vi "Write resource name.vi"(8 "error in (no error)":errorcluster, 10 "RIO Device":T1, 11 "FPGATarget in":refnum<class "FPGATarget.lvclass">) -> (0 "error out":errorcluster, 3 "FPGATarget out":refnum<class "FPGATarget.lvclass">)   [LabVIEW 2013, in "FPGATarget.lvclass"]
uses:
  FPGATarget.lvclass
  <vilib>/userdefined/High Color/nirio_resource_hc.ctl
  FPGATarget.lvclass/FPGATarget.ctl
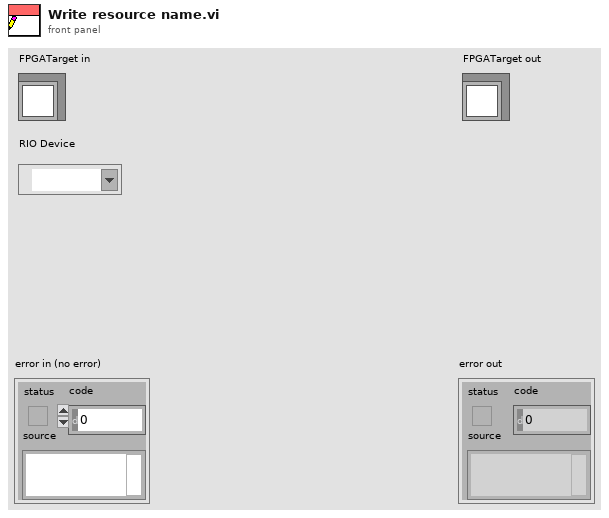
[diagram p1: front panel]
types:
  T1 = typedef "nirio_resource_hc.ctl" = tag
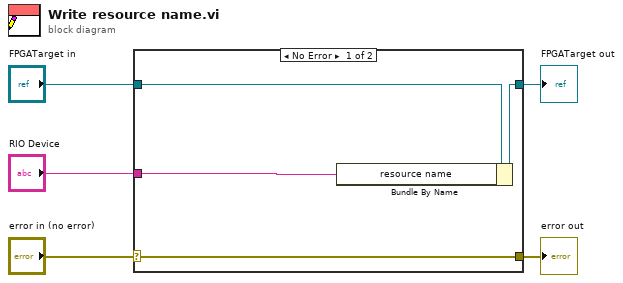
[diagram p0: block diagram]
diagram:
  n1 = case shown="No Error" "error in (no error)" {
    selector: "error in (no error)" -> [w9 w10]
    tunnel: [w9 w10] -> w4
    tunnel: [w7 w11] -> w2
    tunnel: "FPGATarget in" -> [w8 w11]
    tunnel: "RIO Device" -> [w6 _]
    frame No Error {
      n2 = Bundle By Name(cluster=w8, "resource name"=w6) -> (w7:refnum<class "FPGATarget.lvclass">)
    }
    frame Error {
    }
  }
  "error out" <- w4
  "FPGATarget out" <- w2
